vi "Destroy BufferMap.vi"(8 "error in":errorcluster, 9 "Return Elements (T)":bool=TRUE, 11 "Buffer":refnum<data-value>) -> (0 "error out":errorcluster, 2 "elements":refnum<data-value>[](array[refnum]))   [LabVIEW 2013, in "VariantBufferMap.lvclass"]
doc: "This VI releases resources that have been created for the ring buffer."
uses:
  VariantBufferMap.lvclass
  VariantBuffer/VariantBuffer.lvclass
  VariantBufferMap.lvclass/VariantBufferMap.ctl
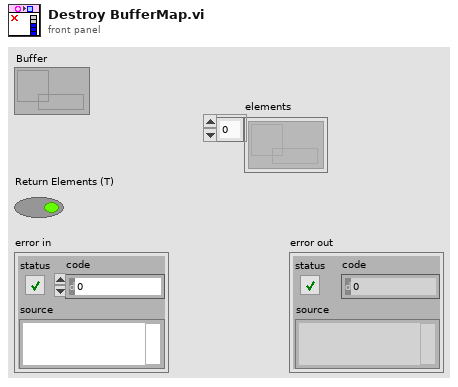
[diagram p1: front panel]
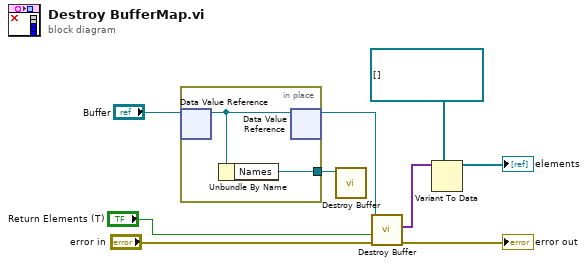
[diagram p0: block diagram]
diagram:
  n1 = in-place {
    in-place-border: [w11] -> w9
    n2 = in-place-dvr #1("Buffer") -> (w10:refnum<class "VariantBufferMap.lvclass">)  [unwired: 1 out]
    n3 = Unbundle By Name(w10) -> ("Names"=w11:refnum<data-value>)
    n4 = in-place-dvr #1(w10) -> (w3:refnum<data-value>)  [unwired: 1 out]
  }
  n5 = call "Destroy Buffer.vi"("Buffer"=w9) -> ()  [unwired: 9 in, 2 out]
  n6 = call "Destroy Buffer.vi"("error in"="error in", "Return Elements (T)"="Return Elements (T)", "Buffer"=w3) -> ("error out"=→"error out":errorcluster, "elements"=w6:variant[])  [unwired: 7 in]
  n7 = Variant To Data(type=refnum<data-value>[] [], Variant=w6) -> (data=→"elements":refnum<data-value>[])  [unwired: 1 in, 1 out]
